vi "Project.vi"() -> ()   [LabVIEW 2022 SP3]
uses:
  <vilib>/DAQmx/read.llb/DAQmx Read (Analog 1D DBL NChan 1Samp).vi
  <vilib>/DAQmx/write.llb/DAQmx Write (Digital Bool 1Line 1Point).vi
  <vilib>/DAQmx/create/channels.llb/DAQmx Create Channel (AI-Voltage-Basic).vi
  <vilib>/DAQmx/create/channels.llb/DAQmx Create Channel (DO-Digital Output).vi
  <vilib>/DAQmx/miscellaneous.llb/DAQmx Fill In Error Info.vi
panel:
  out "FAN":bool
  out "Rain":bool
  out "Fire Alarm":bool
  out "GAS Alarm":bool
  in  "stop":bool
  in  "VISA Refnum in 3":refnum<visa-resource-name>
  in  "VISA Refnum in 2":refnum<visa-resource-name>
  in  "VISA Refnum in":refnum<visa-resource-name>
  out "Real Time Variation of Gas Sensor Output":dbl(graph)
  in  "Buzzer for Gas Sensor":tag
  out "Real Time Temperature Variation":dbl(graph)
  in  "Fan Output":tag
  out "PIR Value":dbl
  out "Motion Detector":bool
  in  "Rain Sensor Output":tag
  out "Rain Sensor Value Indicator":dbl(knob) scale=0.0..6.0
  out "Rain Sensor Value":dbl
  in  "PIR Output for LED Lights":tag
  out "Voltage Value of the temperature sensor":dbl
  out "Temperature Value":dbl
  in  "Thermister Output for Buzzer":tag
  in  "stop 2":bool
  out "Temp Indicator":dbl(knob) scale=0.0..100.0
  out "Voltage Value of the temperature Sensor":dbl(knob) scale=0.0..1.0
  in  "Sensor inputs":tag
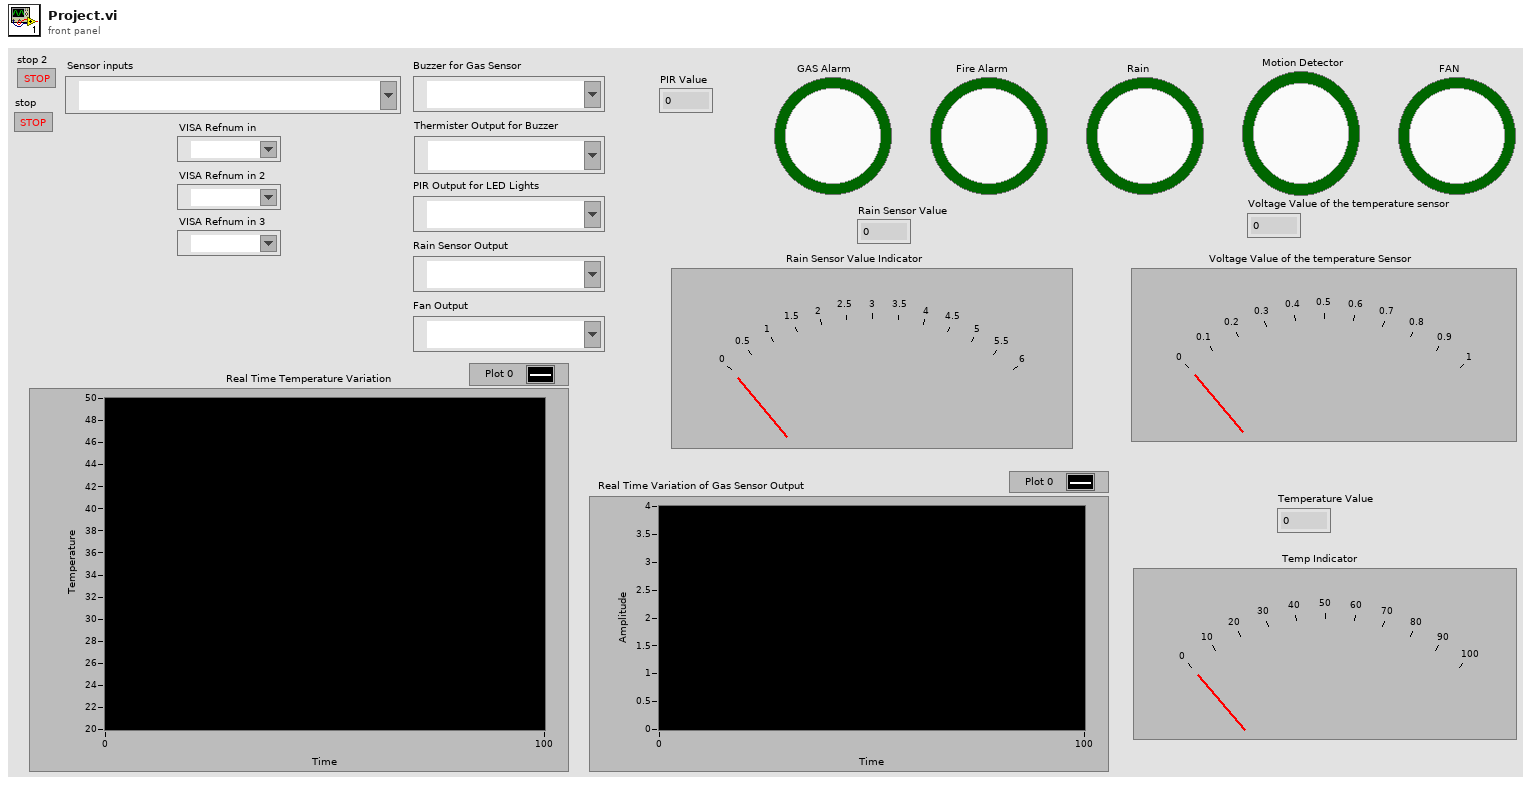
[diagram p1: front panel]
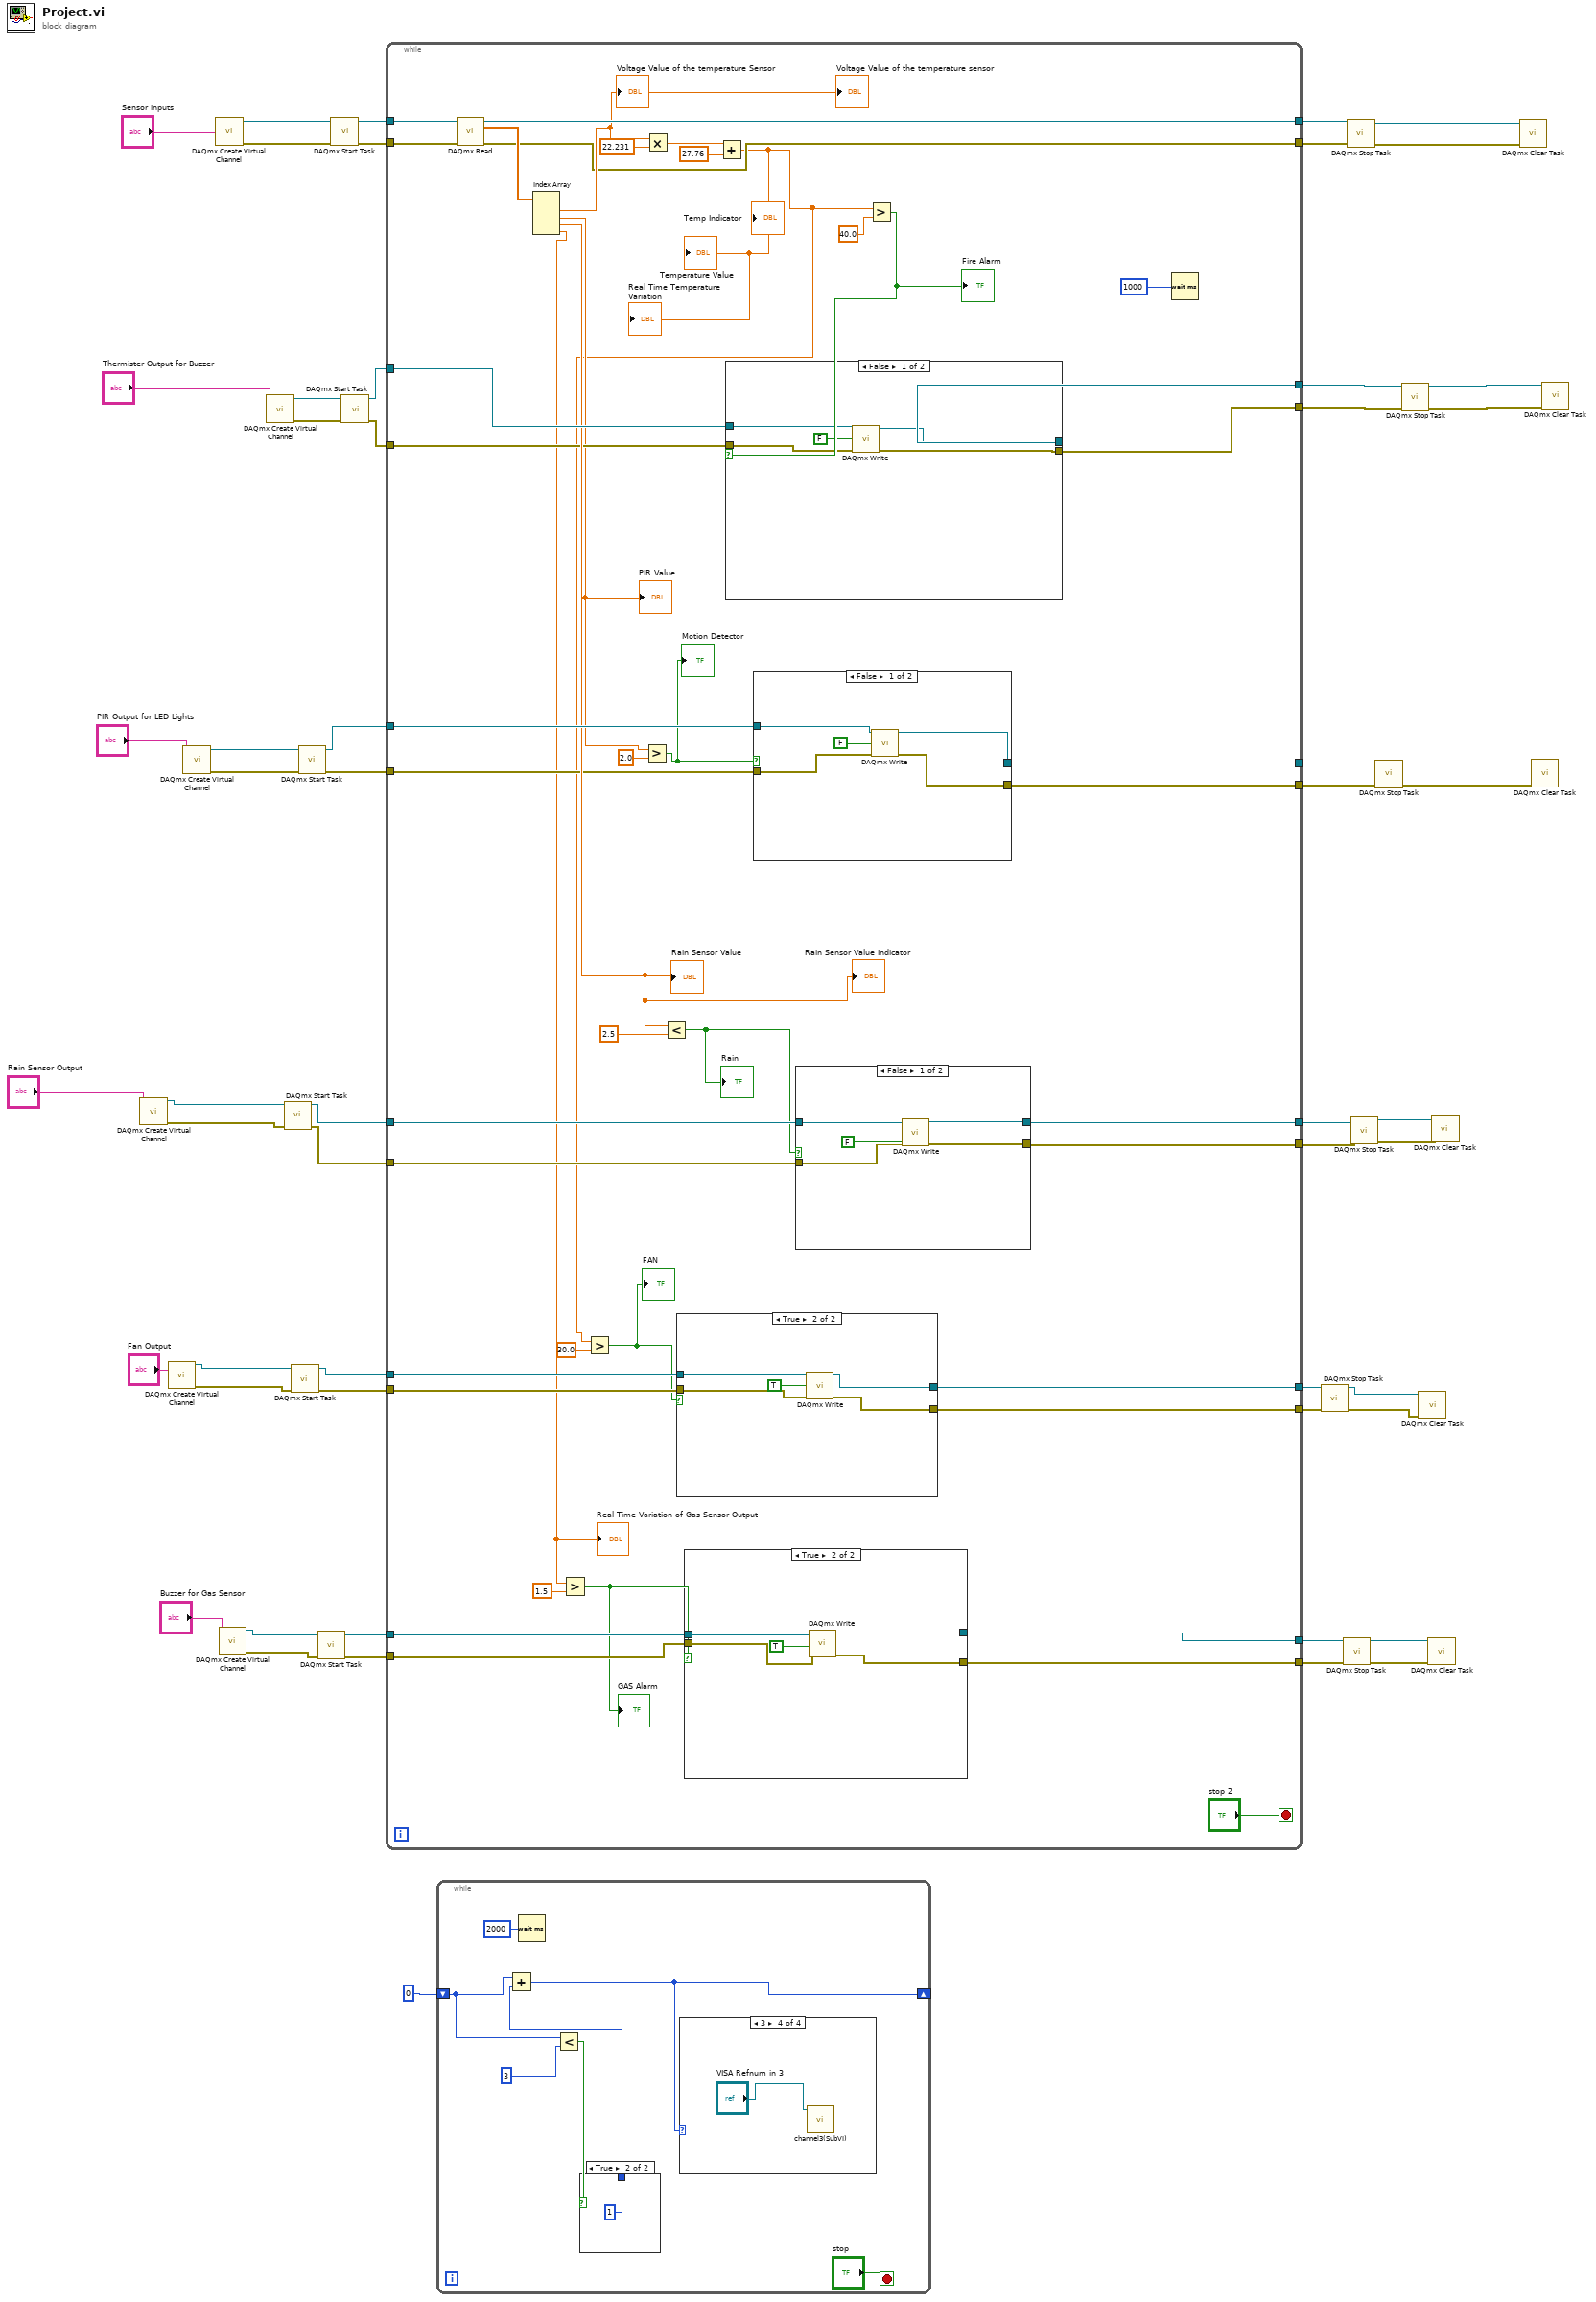
[diagram p0: block diagram]
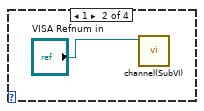
[diagram p3: hidden frame]
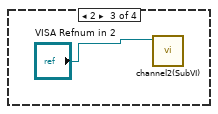
[diagram p4: hidden frame]
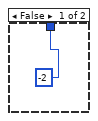
[diagram p5: hidden frame]
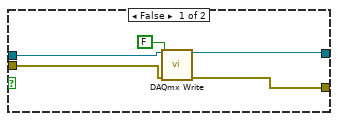
[diagram p6: hidden frame]
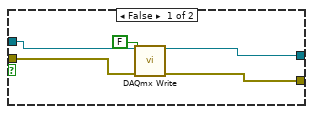
[diagram p7: hidden frame]
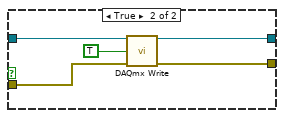
[diagram p8: hidden frame]
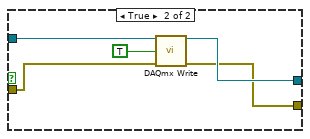
[diagram p9: hidden frame]
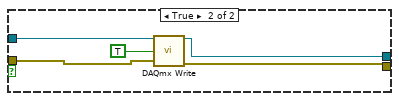
[diagram p10: hidden frame]
diagram:
  n1 = call-poly <vilib>:"DAQmx Create Virtual Channel.vi"("lines"="Rain Sensor Output") -> ("task out"=w39:refnum<k21>, "error out"=w23:errorcluster)  [unwired: 13 in]
  n2 = call-poly <vilib>:"DAQmx Create Virtual Channel.vi"("lines"="Fan Output") -> ("task out"=w19:refnum<k21>, "error out"=w15:errorcluster)  [unwired: 13 in]
  n3 = call-poly <vilib>:"DAQmx Create Virtual Channel.vi"("lines"="PIR Output for LED Lights") -> ("task out"=w44:refnum<k21>, "error out"=w27:errorcluster)  [unwired: 13 in]
  n4 = call-poly <vilib>:"DAQmx Create Virtual Channel.vi"("physical channels"="Sensor inputs") -> ("task out"=w54:refnum<k21>, "error out"=w35:errorcluster)  [unwired: 13 in]
  n5 = call-poly <vilib>:"DAQmx Create Virtual Channel.vi"("lines"="Buzzer for Gas Sensor") -> ("task out"=w9:refnum<k21>, "error out"=w5:errorcluster)  [unwired: 13 in]
  n6 = call-poly <vilib>:"DAQmx Create Virtual Channel.vi"("lines"="Thermister Output for Buzzer") -> ("task out"=w47:refnum<k21>, "error out"=w31:errorcluster)  [unwired: 13 in]
  n7 = call <vilib>:"DAQmx Start Task.vi"("task/channels in"=w39, "error in"=w23) -> ("task out"=w38:refnum<k21>, "error out"=w22:errorcluster)  [unwired: 12 in]
  n8 = call <vilib>:"DAQmx Start Task.vi"("task/channels in"=w19, "error in"=w15) -> ("task out"=w18:refnum<k21>, "error out"=w14:errorcluster)  [unwired: 12 in]
  n9 = call <vilib>:"DAQmx Start Task.vi"("task/channels in"=w44, "error in"=w27) -> ("task out"=w43:refnum<k21>, "error out"=w26:errorcluster)  [unwired: 12 in]
  n10 = call <vilib>:"DAQmx Start Task.vi"("task/channels in"=w9, "error in"=w5) -> ("task out"=w8:refnum<k21>, "error out"=w4:errorcluster)  [unwired: 12 in]
  n11 = call <vilib>:"DAQmx Start Task.vi"("task/channels in"=w54, "error in"=w35) -> ("task out"=w53:refnum<k21>, "error out"=w34:errorcluster)  [unwired: 12 in]
  n12 = call <vilib>:"DAQmx Start Task.vi"("task/channels in"=w47, "error in"=w31) -> ("task out"=w50:refnum<k21>, "error out"=w30:errorcluster)  [unwired: 12 in]
  n13 = while {
    tunnel: w53 -> [w100]
    tunnel: [w99] -> w51
    tunnel: w50 -> [w94]
    tunnel: [w93] -> w49
    tunnel: w43 -> [w90]
    tunnel: [w89] -> w42
    tunnel: w38 -> [w87]
    tunnel: [w86] -> w37
    tunnel: w34 -> [w82]
    tunnel: [w81] -> w33
    tunnel: w30 -> [w80]
    tunnel: [w79] -> w29
    tunnel: w26 -> [w78]
    tunnel: [w77] -> w25
    tunnel: w22 -> [w76]
    tunnel: [w75] -> w21
    tunnel: w18 -> [w71]
    tunnel: [w70] -> w17
    tunnel: w14 -> [w69]
    tunnel: [w68] -> w13
    tunnel: w8 -> [w65]
    tunnel: [w64] -> w7
    tunnel: w4 -> [w63]
    tunnel: [w62] -> w3
    stop <- "stop 2" stop-if-true
    n14 = call-poly <vilib>:"DAQmx Read.vi"("task/channels in"=w100, "error in"=w82) -> ("task out"=w99:refnum<k21>, "data"=w85:dbl[], "error out"=w81:errorcluster)  [unwired: 11 in]
    n15 = Index Array(array=w85) -> (element #1=w84:dbl, element #2=w72:dbl, element #3=w83:dbl, element #4=w60:dbl)  [unwired: 4 in]
    "Voltage Value of the temperature Sensor" <- w84
    "Voltage Value of the temperature sensor" <- w84
    "Rain Sensor Value" <- w83
    "Rain Sensor Value Indicator" <- w83
    "PIR Value" <- w72
    "Real Time Variation of Gas Sensor Output" <- w60
    n16 = Greater?(x=w60, y=1.5) -> (0:w57:bool)
    "GAS Alarm" <- w57
    n17 = Greater?(x=w72, y=2.0) -> (0:w73:bool)
    "Motion Detector" <- w73
    n18 = Multiply(x=w84, y=22.231) -> (x*y=w97:dbl)
    n19 = Less?(x=w83, y=2.5) -> (x < y?=w59:bool)
    "Rain" <- w59
    n20 = case shown="True" w57 {
      tunnel: w65 -> [w105 w109]
      tunnel: [w104 w108] -> w64
      tunnel: w63 -> [w103 w107]
      tunnel: [w102 w106] -> w62
      frame False {
        n21 = call-poly <vilib>:"DAQmx Write.vi"("task/channels in"=w105, "data"=FALSE, "error in"=w103) -> ("task out"=w104:refnum<k21>, "error out"=w102:errorcluster)  [unwired: 10 in, 1 out]
      }
      frame True {
        n22 = call-poly <vilib>:"DAQmx Write.vi"("task/channels in"=w109, "data"=TRUE, "error in"=w107) -> ("task out"=w108:refnum<k21>, "error out"=w106:errorcluster)  [unwired: 10 in, 1 out]
      }
    }
    n23 = Add(x=w97, y=27.76) -> (x+y=w66:dbl)
    "Temp Indicator" <- w66
    "Temperature Value" <- w66
    "Real Time Temperature Variation" <- w66
    n24 = Greater?(x=w66, y=30.0) -> (0:w56:bool)
    "FAN" <- w56
    n25 = case shown="True" w56 {
      tunnel: w71 -> [w115 w120]
      tunnel: [w114 w119] -> w70
      tunnel: w69 -> [w113 w118]
      tunnel: [w112 w117] -> w68
      frame False {
        n26 = call-poly <vilib>:"DAQmx Write.vi"("task/channels in"=w115, "data"=FALSE, "error in"=w113) -> ("task out"=w114:refnum<k21>, "error out"=w112:errorcluster)  [unwired: 10 in, 1 out]
      }
      frame True {
        n27 = call-poly <vilib>:"DAQmx Write.vi"("task/channels in"=w120, "data"=TRUE, "error in"=w118) -> ("task out"=w119:refnum<k21>, "error out"=w117:errorcluster)  [unwired: 10 in, 1 out]
      }
    }
    n28 = case shown="False" w73 {
      tunnel: w90 -> [w135 w139]
      tunnel: [w134 w138] -> w89
      tunnel: w78 -> [w132 w137]
      tunnel: [w131 w136] -> w77
      frame False {
        n29 = call-poly <vilib>:"DAQmx Write.vi"("task/channels in"=w135, "data"=FALSE, "error in"=w132) -> ("task out"=w134:refnum<k21>, "error out"=w131:errorcluster)  [unwired: 10 in, 1 out]
      }
      frame True {
        n30 = call-poly <vilib>:"DAQmx Write.vi"("task/channels in"=w139, "data"=TRUE, "error in"=w137) -> ("task out"=w138:refnum<k21>, "error out"=w136:errorcluster)  [unwired: 10 in, 1 out]
      }
    }
    n31 = case shown="False" w59 {
      tunnel: w87 -> [w124 w129]
      tunnel: [w123 w128] -> w86
      tunnel: w76 -> [w122 w127]
      tunnel: [w121 w126] -> w75
      frame False {
        n32 = call-poly <vilib>:"DAQmx Write.vi"("task/channels in"=w124, "data"=FALSE, "error in"=w122) -> ("task out"=w123:refnum<k21>, "error out"=w121:errorcluster)  [unwired: 10 in, 1 out]
      }
      frame True {
        n33 = call-poly <vilib>:"DAQmx Write.vi"("task/channels in"=w129, "data"=TRUE, "error in"=w127) -> ("task out"=w128:refnum<k21>, "error out"=w126:errorcluster)  [unwired: 10 in, 1 out]
      }
    }
    n34 = Greater?(x=w66, y=40.0) -> (0:w58:bool)
    "Fire Alarm" <- w58
    n35 = case shown="False" w58 {
      tunnel: w94 -> [w143 w150]
      tunnel: [w144 w149] -> w93
      tunnel: w80 -> [w142 w147]
      tunnel: [w141 w146] -> w79
      frame False {
        n36 = call-poly <vilib>:"DAQmx Write.vi"("task/channels in"=w143, "data"=FALSE, "error in"=w142) -> ("task out"=w144:refnum<k21>, "error out"=w141:errorcluster)  [unwired: 10 in, 1 out]
      }
      frame True {
        n37 = call-poly <vilib>:"DAQmx Write.vi"("task/channels in"=w150, "data"=TRUE, "error in"=w147) -> ("task out"=w149:refnum<k21>, "error out"=w146:errorcluster)  [unwired: 10 in, 1 out]
      }
    }
    n38 = Wait (ms)(milliseconds to wait=u32 1000) -> ()  [unwired: 1 out]
  }
  n39 = while {
    shift-right: [w151] -> _
    shift-left: 0 -> [w156]
    stop <- "stop" stop-if-true
    n40 = Wait (ms)(milliseconds to wait=u32 2000) -> ()  [unwired: 1 out]
    n41 = Less?(x=w156, y=3) -> (x < y?=w154:bool)
    n42 = case shown="True" w154 {
      tunnel: [-2 1] -> w153
      frame False {
      }
      frame True {
      }
    }
    n43 = Add(x=w156, y=w153) -> (x+y=w151:i32)
    n44 = case shown="3" w151 {
      frame 0, Default {
      }
      frame 1 {
        n45 = call "channel(SubVI).vi"("VISA Refnum in"="VISA Refnum in") -> ()  [unwired: 11 in]
      }
      frame 2 {
        n46 = call "channel2(SubVI).vi"("VISA Refnum in"="VISA Refnum in 2") -> ()  [unwired: 11 in]
      }
      frame 3 {
        n47 = call "channel3(SubVI).vi"("VISA Refnum in"="VISA Refnum in 3") -> ()  [unwired: 11 in]
      }
    }
  }
  n48 = call <vilib>:"DAQmx Stop Task.vi"("task/channels in"=w17, "error in"=w13) -> ("task out"=w16:refnum<k21>, "error out"=w12:errorcluster)  [unwired: 12 in]
  n49 = call <vilib>:"DAQmx Stop Task.vi"("task/channels in"=w7, "error in"=w3) -> ("task out"=w6:refnum<k21>, "error out"=w2:errorcluster)  [unwired: 12 in]
  n50 = call <vilib>:"DAQmx Stop Task.vi"("task/channels in"=w51, "error in"=w33) -> ("task out"=w52:refnum<k21>, "error out"=w32:errorcluster)  [unwired: 12 in]
  n51 = call <vilib>:"DAQmx Stop Task.vi"("task/channels in"=w37, "error in"=w21) -> ("task out"=w36:refnum<k21>, "error out"=w20:errorcluster)  [unwired: 12 in]
  n52 = call <vilib>:"DAQmx Stop Task.vi"("task/channels in"=w42, "error in"=w25) -> ("task out"=w41:refnum<k21>, "error out"=w24:errorcluster)  [unwired: 12 in]
  n53 = call <vilib>:"DAQmx Stop Task.vi"("task/channels in"=w49, "error in"=w29) -> ("task out"=w48:refnum<k21>, "error out"=w28:errorcluster)  [unwired: 12 in]
  n54 = call <vilib>:"DAQmx Clear Task.vi"("task in"=w16, "error in"=w12) -> ()  [unwired: 13 in, 1 out]
  n55 = call <vilib>:"DAQmx Clear Task.vi"("task in"=w6, "error in"=w2) -> ()  [unwired: 13 in, 1 out]
  n56 = call <vilib>:"DAQmx Clear Task.vi"("task in"=w36, "error in"=w20) -> ()  [unwired: 13 in, 1 out]
  n57 = call <vilib>:"DAQmx Clear Task.vi"("task in"=w52, "error in"=w32) -> ()  [unwired: 13 in, 1 out]
  n58 = call <vilib>:"DAQmx Clear Task.vi"("task in"=w41, "error in"=w24) -> ()  [unwired: 13 in, 1 out]
  n59 = call <vilib>:"DAQmx Clear Task.vi"("task in"=w48, "error in"=w28) -> ()  [unwired: 13 in, 1 out]
